vi "Gui_SetupLoops.vi"(8 "error in (no error)":errorcluster, 11 "Variant":variant) -> (0 "error out":errorcluster caption="sortie d'erreur", 3 "Variant Output":variant)   [LabVIEW 2024]
doc: "This VI setup the LOOPS parameters. (Only OPO parameters at this moment).\n\n1. The EXPERT parameters are passed through a Variant as input.\n2. Init the controls with the previous values.\n3. Wait for the user events, and update controls accordingly.\n4. When OK is pushed, the last values of the controls are stored into Variant."
uses:
  controls/LOOPS_Inputs.ctl
  controls/OPO_Inputs.ctl
panel:
  in  "OPO Inputs":T1={"OPO AutoAlignment ON"=FALSE, "OPO Start Value"=210.0, "OPO Stop Value"=270.0, "OPO Step"=30.0} {"OPO Step" min=0.5 max=60.0 format="%#.1f"; "OPO Stop Value" min=210.0 max=270.0 format="%#.1f"; "OPO Start Value" min=210.0 max=270.0 format="%#.1f"}
  out "OPO Values":dbl[](array[numeric]) format="%#.1f"
  out "Number of Loops":i16
  in  "OK":bool
  in  "LOOPS Inputs":T2={"Number of Loops"=0, "Loop Current Value"=0, "OPO Inputs"={"OPO AutoAlignment ON"=FALSE, "OPO Start Value"=210.0, "OPO Stop Value"=270.0, "OPO Step"=10.0}} {"OPO Inputs"."OPO Step" min=0.5 max=60.0 format="%#.1f"; "OPO Inputs"."OPO Stop Value" min=210.0 max=270.0 format="%#.1f"; "OPO Inputs"."OPO Start Value" min=210.0 max=270.0 format="%#.1f"}
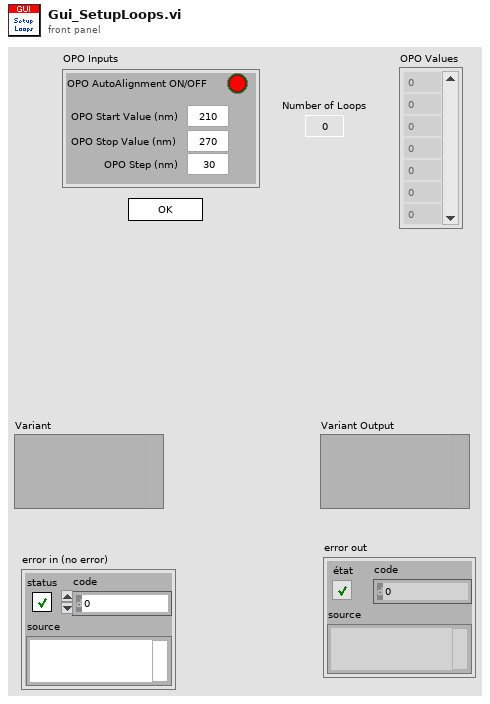
[diagram p1: front panel]
types:
  T1 = typedef "OPO_Inputs.ctl" = cluster{"OPO AutoAlignment ON":bool, "OPO Start Value":dbl, "OPO Stop Value":dbl, "OPO Step":dbl}
  T2 = typedef "LOOPS_Inputs.ctl" = cluster{"Number of Loops":i16, "Loop Current Value":i16, "OPO Inputs":T1}
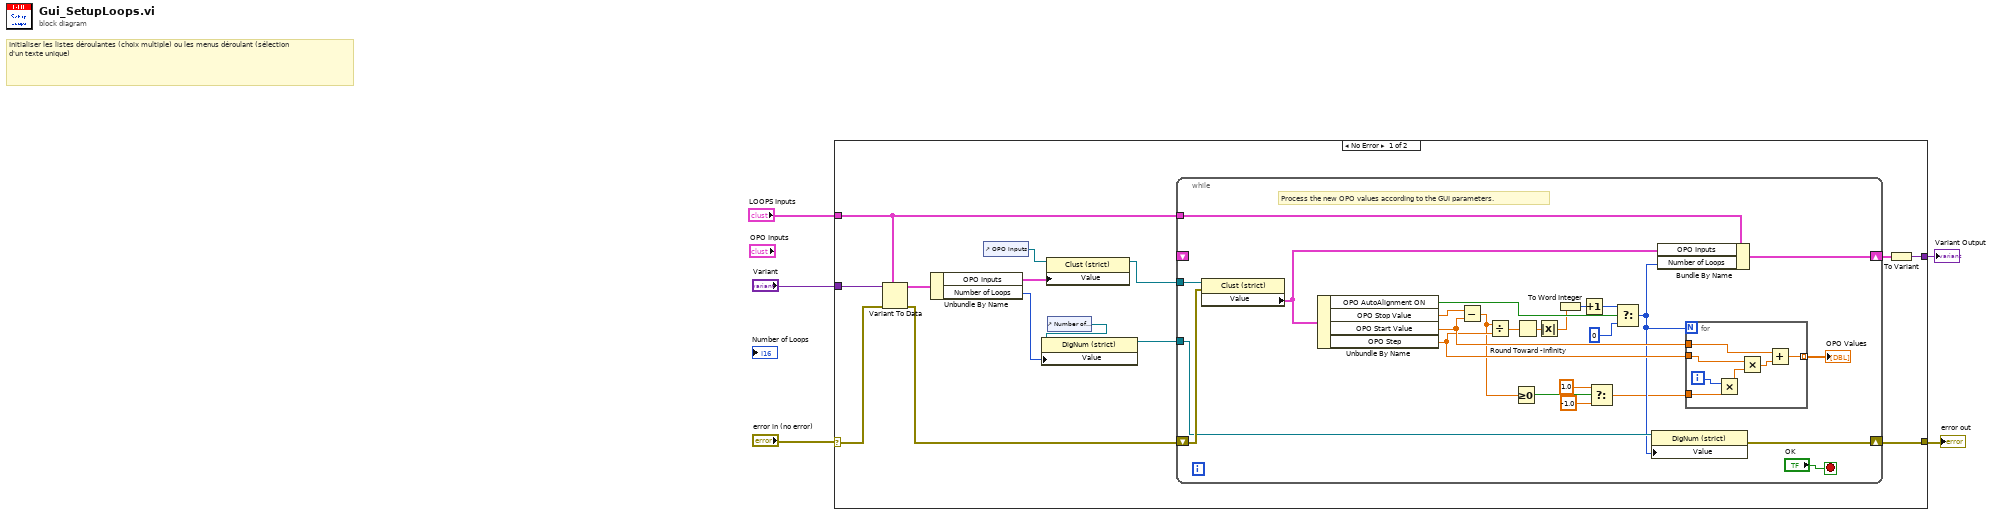
[diagram p0: block diagram]
diagram:
  # "Initialiser les listes déroulantes (choix multiple) ou les menus déroulant (sélection d'un texte unique)"
  n1 = case shown="No Error" "error in (no error)" {
    selector: "error in (no error)" -> [w18 w53]
    tunnel: [w19 w52] -> w3
    tunnel: "Variant" -> [w17 w52]
    tunnel: "LOOPS Inputs" -> [w8 _]
    tunnel: [w11 w53] -> w1
    frame No Error {
      n2 = Variant To Data(error in=w18, type=w8, Variant=w17) -> (data=w16:T2, error out=w9:errorcluster)
      n3 = Unbundle By Name(w16) -> ("OPO Inputs"=w15:T1, "Number of Loops"=w10:i16)
      n4 = control-ref of="OPO Inputs"() -> (w6:refnum<vi>)
      n5 = property class="Clust (strict)"(reference=w6, "Value"=w15) -> (reference out=w13:refnum<vi>)  [unwired: 1 in, 1 out]
      n6 = control-ref of="Number of Loops"() -> (w14:refnum<vi>)
      n7 = property class="DigNum (strict)"(reference=w14, "Value"=w10) -> (reference out=w12:refnum<vi>)  [unwired: 1 in, 1 out]
      n8 = while {
        tunnel: w13 -> [w43]
        tunnel: w12 -> [w33]
        shift-right: [w42] -> w7
        shift-left: _ -> [_]
        shift-right: [w32] -> w11
        shift-left: w9 -> [w34]
        tunnel: w8 -> [w30]
        stop <- "OK" stop-if-true
        # "Process the new OPO values according to the GUI parameters."
        n9 = property class="Clust (strict)"(reference=w43, error in=w34) -> ("Value"=w41:T1)  [unwired: 2 out]
        n10 = Unbundle By Name(w41) -> ("OPO AutoAlignment ON"=w38:bool, "OPO Stop Value"=w40:dbl, "OPO Start Value"=w29:dbl, "OPO Step"=w28:dbl)
        n11 = Subtract(x=w40, y=w29) -> (x-y=w24:dbl)
        n12 = Divide(x=w24, y=w28) -> (x/y=w39:dbl)
        n13 = Greater Or Equal To 0?(x=w24) -> (x >= 0?=w23:bool)
        n14 = Round Toward -Infinity(1:w39) -> (0:w36:dbl)
        n15 = Absolute Value(x=w36) -> (abs(x)=w25:dbl)
        n16 = To Word Integer(number=w25) -> (16bit integer=w35:i16)
        n17 = Increment(x=w35) -> (x+1=w31:i16)
        n18 = Select(t=1.0, s=w23, f=-1.0) -> (s? t:f=w20:dbl)
        n19 = Select(t=w31, s=w38, f=i16 0) -> (s? t:f=w27:i16)
        n20 = property class="DigNum (strict)"(reference=w33, "Value"=w27) -> (error out=w32:errorcluster)  [unwired: 1 in, 1 out]
        n21 = Bundle By Name(cluster=w30, "OPO Inputs"=w41, "Number of Loops"=w27) -> (w42:T2)
        n22 = for {
          N: w27 -> [_]
          tunnel: w29 -> [w49]
          tunnel: w28 -> [w51]
          tunnel: [w48] -> w26 mode=indexing
          tunnel: w20 -> [w46]
          i -> [w45]
          n23 = Multiply(x=w45, y=w46) -> (x*y=w47:dbl)
          n24 = Multiply(x=w51, y=w47) -> (x*y=w50:dbl)
          n25 = Add(x=w49, y=w50) -> (x+y=w48:dbl)
        }
        "OPO Values" <- w26
      }
      n26 = To Variant(anything=w7) -> (Variant=w19:variant)
    }
    frame Error {
    }
  }
  "error out" <- w1
  "Variant Output" <- w3
